vi "PH_ImageCalibrator.contents.vi"   [LabVIEW 2014, in "PH_ImageCalibrator.lvlib"]
doc: "This class takes and stores several beam profile settings. This is relevant for the class PH_ImageOperator.\n\nThis class is part of the PHELIX user layer."
uses:
  PH_ImageCalibrator.lvlib
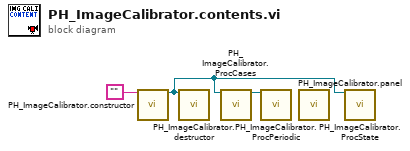
[diagram p0: block diagram]
diagram:
  n1 = call "PH_ImageCalibrator.constructor.vi"("name"="") -> ("i ref out"=w1:refnum<vi>)  [unwired: 16 in, 2 out]
  n2 = call "PH_ImageCalibrator.destructor.vi"("i ref in"=w1) -> ()  [unwired: 18 in, 1 out]
  n3 = call "PH_ImageCalibrator.ProcCases.vi"("i ref in"=w1) -> ("i ref out"=w3:refnum<vi>)  [unwired: 16 in, 2 out]
  n4 = call "PH_ImageCalibrator.ProcPeriodic.vi"("i ref in"=w3) -> ()  [unwired: 16 in, 3 out]
  n5 = call "PH_ImageCalibrator.panel.vi"() -> ()  [unwired: 19 in, 1 out]
  n6 = call "PH_ImageCalibrator.ProcState.vi"("i ref in"=w1) -> ()  [unwired: 16 in, 3 out]
